vi "_Translate Leybold Message.vi"(11 "LeyboldMessage":string="\u0002\u0016\u0000\u0010\u0003\u0000\u0000\u0000\u0000\u0000j‹\u0014\u0000j\u0000 \u0000]\u0000(\u0000\u0018Õ") -> (0 "Voltage":u16=35604, 1 "Current":dbl=35604.0, 2 "Temperature":u16=35604, 3 "Frequency":u16=35604, 4 "Byte11&12":u16=35604 format="%04x", 5 "Pump Status":bool[](array[boolean])=[TRUE, FALSE, FALSE, FALSE, TRUE, FALSE, TRUE, TRUE, FALSE, FALSE, FALSE, TRUE, FALSE, TRUE, FALSE, FALSE], 6 "Error":string, 7 "Parameter":u32=35604)   [LabVIEW 2015]
panel:
  out "Telegram (24 bytes in Hex)":u8[](array[numeric])=[2, 22, 0, 16, 3, 0, 0, 0, 0, 0, 106, 139, 20, 0, 106, 0, 32, 0, 93, 0, 40, 0, 24, 213] format="%02x"
  # "bit-15, Process channel enabled"
  # "bit-14, Collective warning"
  # "bit-13, Overload warning"
  # "bit-12, No function"
  # "bit-11, Pump is turning"
  # "byte-0"
  # "byte-23"
  # "bit-10, Normal operation detained"
  # "bit-9, Parameter channel enabled"
  # "bit-8, No function"
  # "bit-7, Temperature warning"
  # "bit-6, Switch-on lock"
  # "bit-5, Decelerating"
  # "bit-4, Accelerating"
  # "bit-3, Error condition (all components)"
  # "bit-2, Operation enabled"
  # "bit-1, No function"
  # "bit-0, Ready for operation"
  # "(in Hex for byte 11&12)"
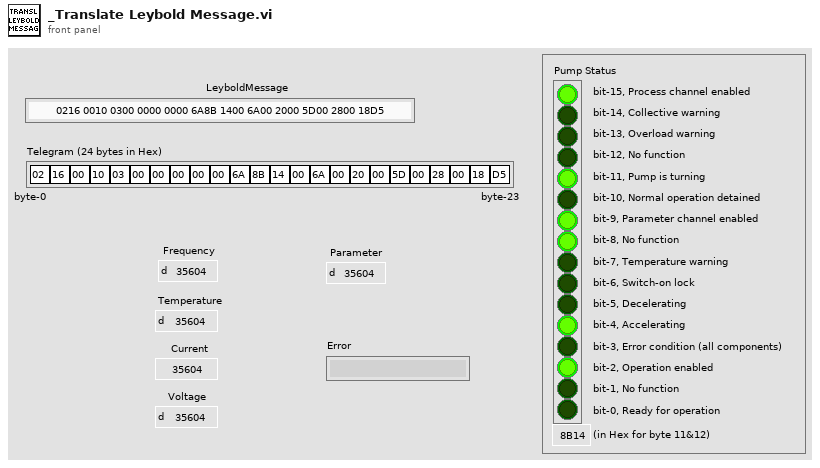
[diagram p1: front panel]
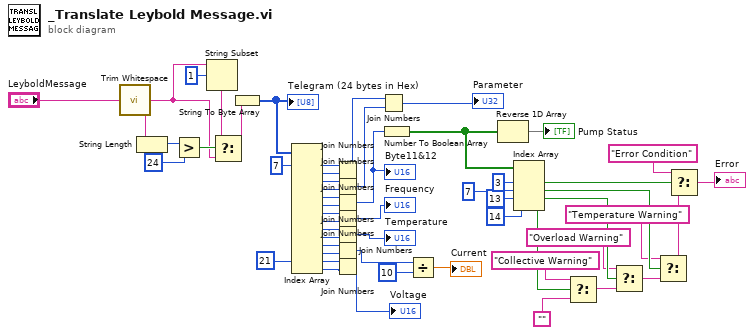
[diagram p0: block diagram]
diagram:
  n1 = call <vilib>:"Trim Whitespace.vi"("string"="LeyboldMessage") -> ("trimmed string"=w2:string)  [unwired: 1 in]
  n2 = String Length(string=w2) -> (length=w7:i32)
  n3 = Greater?(x=w7, y=24) -> (0:w5:bool)
  n4 = String Subset(string=w2, offset (0)=1) -> (substring=w1:string)  [unwired: 1 in]
  n5 = Select(t=w1, s=w5, f=w2) -> (s? t:f=w3:string)
  n6 = String To Byte Array(string=w3) -> (unsigned byte array=w53:u8[])
  "Telegram (24 bytes in Hex)" <- w53
  n7 = Index Array(array=w53, index #1=7 ("index"), index #13=21 ("index")) -> (element #1=w51:u8, element #2=w47:u8, element #3=w49:u8, element #4=w46:u8, element #5=w48:u8, element #6=w45:u8, element #7=w44:u8, element #8=w43:u8, element #9=w40:u8, element #10=w39:u8, element #11=w38:u8, element #12=w37:u8, element #13=w35:u8, element #14=w34:u8)  [unwired: 12 in]
  n8 = Join Numbers(hi=w51, lo=w47) -> ((hi.lo)=w28:u16)
  n9 = Join Numbers(hi=w49, lo=w46) -> ((hi.lo)=w27:u16)
  n10 = Join Numbers(hi=w48, lo=w45) -> ((hi.lo)=w29:u16)
  "Byte11&12" <- w29
  n11 = Join Numbers(hi=w44, lo=w43) -> ((hi.lo)=→"Frequency":u16)
  n12 = Join Numbers(hi=w40, lo=w39) -> ((hi.lo)=→"Temperature":u16)
  n13 = Join Numbers(hi=w38, lo=w37) -> ((hi.lo)=w32:u16)
  n14 = Join Numbers(hi=w35, lo=w34) -> ((hi.lo)=→"Voltage":u16)
  n15 = Join Numbers(hi=w28, lo=w27) -> ((hi.lo)=→"Parameter":u32)
  n16 = Number To Boolean Array(number=w29) -> (Boolean array=w22:bool[])
  n17 = Divide(x=w32, y=u16 10) -> (x/y=→"Current":dbl)
  n18 = Reverse 1D Array(array=w22) -> (reversed array=→"Pump Status":bool[])
  n19 = Index Array(array=w22, index #1=3 ("index"), index #2=7 ("index"), index #3=13 ("index"), index #4=14 ("index")) -> (element #1=w20:bool, element #2=w18:bool, element #3=w13:bool, element #4=w17:bool)
  n20 = Select(t="Collective Warning", s=w17, f="") -> (s? t:f=w14:string)
  n21 = Select(t="Overload Warning", s=w13, f=w14) -> (s? t:f=w12:string)
  n22 = Select(t="Temperature Warning", s=w18, f=w12) -> (s? t:f=w9:string)
  n23 = Select(t="Error Condition", s=w20, f=w9) -> (s? t:f=→"Error":string)
